vi "Read Gyro.vi"() -> ()   [LabVIEW 2015]
uses:
  <vilib>/Platform/TimedLoop/XDataNode/timing_clust.ctl
  <vilib>/Platform/TimedLoop/XDataNode/nitl_modes.ctl
  <vilib>/Platform/TimedLoop/XDataNode/wakeup.ctl
  <vilib>/FPGAPlugInAG/myRIO-1900/niLvFpga_Open_myRIO-1900.vi
  <vilib>/rvi/interface/common/dynamic/niFpgaDynamicAddResources.vi
  <vilib>/Utility/error.llb/Error Cluster From Error Code.vi
  <vilib>/rvi/errors/niLvFpgaAdjustHostInterfaceError.vi
  <vilib>/rvi/interface/nirviOpenFPGA/nirviOpenFPGA.xnode
  FPGA Bitfiles/Milestone4_FPGATarget_FPGA_pNQ72xw5+dw.lvbitx
  FPGA.vi
  <vilib>/rvi/interface/nirviReadWriteControl/nirviReadWriteControl.xnode
  <vilib>/platform/TimedLoop/XDataNode/XDataNode.xnode
  <vilib>/Platform/TimedLoop/XDataNode/XDNodeRunTimeDep.lvlib
  NiFpgaLv.dll
  <vilib>/rvi/interface/Simulation/niFpgaSimulationCallBeginRW.vi
panel:
  out "Data bit array":bool[](array[boolean])
  out "Numeric":i32
  in  "stop":bool
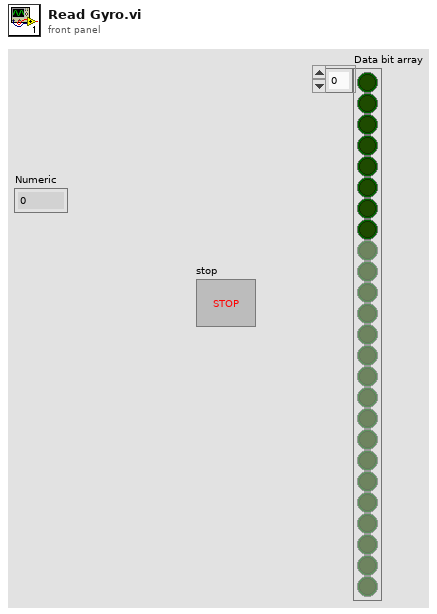
[diagram p1: front panel]
types:
  T1 = typedef "XDNodeRunTimeDep.lvlib/timing_clust.ctl" = cluster{"Expected End [f-1]":u64, "Actual End [f-1]":u64, "Finished Late? [f-1]":bool, "Expected End [i-1]":u64, "Actual End [i-1]":u64, "Finished Late? [i-1]":bool, "Expected Start [i]":u64, "Actual Start [i]":u64, "Expected Start [f]":u64, "Actual Start [f]":u64, "Source Name":string, "Structure Name":string, "Period":i64, "Deadline":i64, "Offset":i64, "Start":i64, "Priority":i32, "Timeout":i32, "Mode":T2, "Wakeup Reason":T3, "Error":errorcluster, "Source Type":string, "Secondary Source Type":string, "Global End Time":u64, "Global Start Time":u64, "Frame Duration":u64, "Iteration Duration":u64, "Assigned CPU":i32, "I/O Scan Engine Mode":u32}
  T2 = typedef "XDNodeRunTimeDep.lvlib/nitl_modes.ctl" = enum32{"No Change", "Process missed periods, maintain original phase", "Discard missed periods, maintain original phase", "Process missed periods, ignore original phase", "Discard missed periods, ignore original phase"}
  T3 = typedef "XDNodeRunTimeDep.lvlib/wakeup.ctl" = enum32{"Normal", "Aborted", "Asynchronous wakeup", "Timing source error", "Timed loop error", "Timeout"}
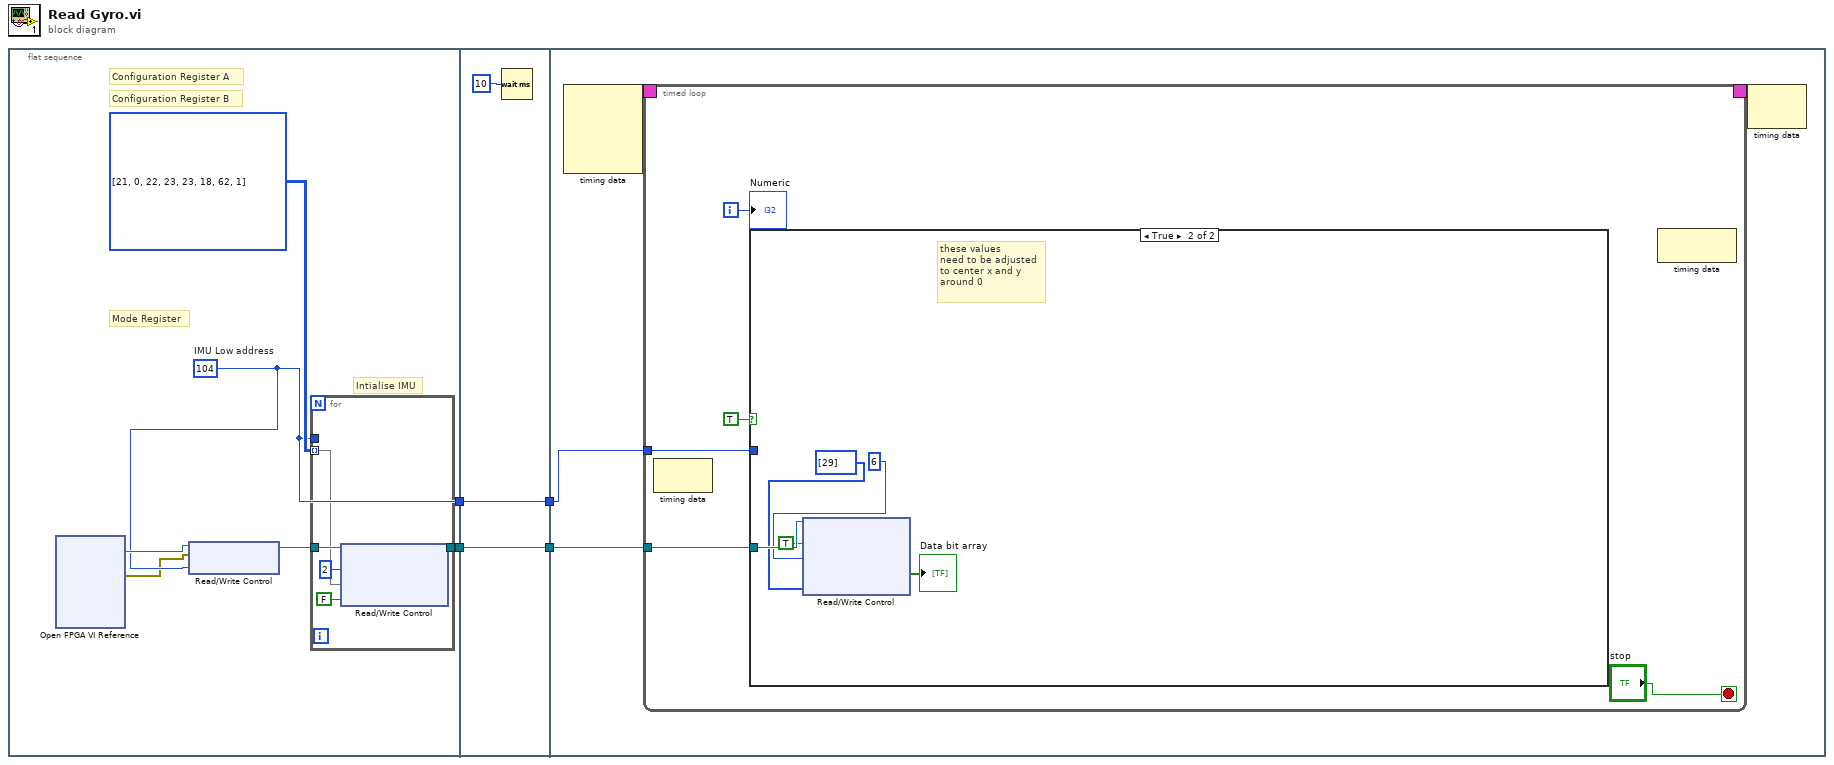
[diagram p0: block diagram]
diagram:
  n1 = flat-sequence {
    tunnel: [w7] -> w4
    tunnel: [w6] -> w2
    tunnel: w4 -> [w18]
    tunnel: [w18] -> w3
    tunnel: w2 -> [w16]
    tunnel: [w16] -> w1
    tunnel: w3 -> [w20]
    tunnel: w1 -> [w19]
    frame #0 {
      w7 = u8 104  # IMU Low address
      # "Mode Register"
      # "Intialise IMU"
      # "Configuration Register B"
      # "Configuration Register A"
      n2 = xnode "Open FPGA VI Reference"() -> ("FPGA VI Reference Out"=w9:refnum<k20>, "error out"=w5:errorcluster)  [unwired: 2 in]
      n3 = xnode "Read/Write Control"("FPGA VI Reference In"=w9, "error in"=w5, "Slave Address"=w7) -> ("FPGA VI Reference Out"=w8:refnum<k20>)  [unwired: 1 out]
      n4 = for {
        tunnel: i8[][] [[21, 0], [22, 23], [23, 18], [62, 1]] -> [w14] mode=indexing
        tunnel: w7 -> [_]
        tunnel: w8 -> [w15]
        tunnel: [w12] -> w6
        n5 = xnode "Read/Write Control"("FPGA VI Reference In"=w15, "Number of bytes"=i16 2, "Data to send"=w14, "Read"=FALSE) -> ("FPGA VI Reference Out"=w12:refnum<k20>)  [unwired: 1 in, 1 out]
      }
    }
    frame #1 {
      n6 = Wait (ms)(milliseconds to wait=u32 10) -> ()  [unwired: 1 out]
    }
    frame #2 {
      n7 = node-c288() -> (w22:T1)  [unwired: 4 in]
      n8 = timed-loop {
        timing: w22 -> [_]
        timing-out: [_] -> w21
        tunnel: w20 -> [w27]
        tunnel: w19 -> [w23]
        i -> [w25]
        stop <- "stop" stop-if-true
        n9 = node-c288() -> ()  [unwired: 1 in, 1 out]
        n10 = case shown="True" TRUE {
          tunnel: w27 -> [_ _]
          tunnel: w23 -> [_ w32]
          frame False {
          }
          frame True {
            # "these values\nneed to be adjusted\nto center x and y\naround 0"
            n11 = xnode "Read/Write Control"("FPGA VI Reference In"=w32, "Read"=TRUE, "Number of bytes"=u32 6 ("Byte Count"), "Data to send"=u8[] [29] ("Bytes to Write")) -> ("Data bit array"=→"Data bit array":bool[])  [unwired: 1 in, 2 out]
          }
        }
        n12 = node-c288() -> ()  [unwired: 1 in, 1 out]
        "Numeric" <- w25
      }
      n13 = node-c288(w21) -> ()  [unwired: 1 out]
    }
  }
